vi "Check Refnum.vi"(11 "Msg EnQ in":refnum<class "Msg EnQ.lvclass">) -> (2 "Msg EnQ out":refnum<class "Msg EnQ.lvclass">)   [LabVIEW 2021, in "AAM.lvlib" / "Msg EnQ.lvclass"]
uses:
  Msg EnQ.lvclass
  Normal Msg EnQ/Normal Msg EnQ.lvclass
  C:/PPLs/LabVIEW-Composed-Actor-Model-LVCAM/LabVIEW-Composed-Actor-Model-LVCAM/AAM/AAM/Msg EnQ/Msg EnQ.lvclass
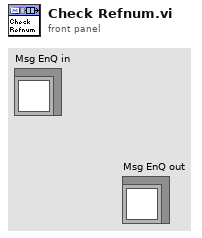
[diagram p1: front panel]
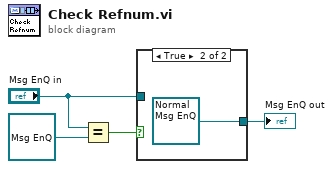
[diagram p0: block diagram]
diagram:
  n1 = Equal?(x="Msg EnQ in", y=refnum<class "Msg EnQ.lvclass"> refnum) -> (x = y?=w3:bool)
  n2 = case shown="True" w3 {
    tunnel: "Msg EnQ in" -> [w5 _]
    tunnel: [w5 refnum<class "Normal Msg EnQ.lvclass"> refnum ("AAM.lvlib:Normal Msg EnQ.lvclass")] -> w1
    frame False {
    }
    frame True {
    }
  }
  "Msg EnQ out" <- w1
